vi "Postion Sub.vi"(11 "inpute":string) -> (2 "pos":string, 3 "数字":u32)   [LabVIEW 2015]
panel:
  out "连接的字符串 3":string
  out "子字符串 8":string
  out "子字符串 7":string
  out "子字符串 6":string
  out "连接的字符串 2":string
  out "连接的字符串":string
  out "子字符串 5":string
  out "子字符串 4":string
  out "子字符串 3":string
  out "子字符串 2":string
  out "子字符串":string
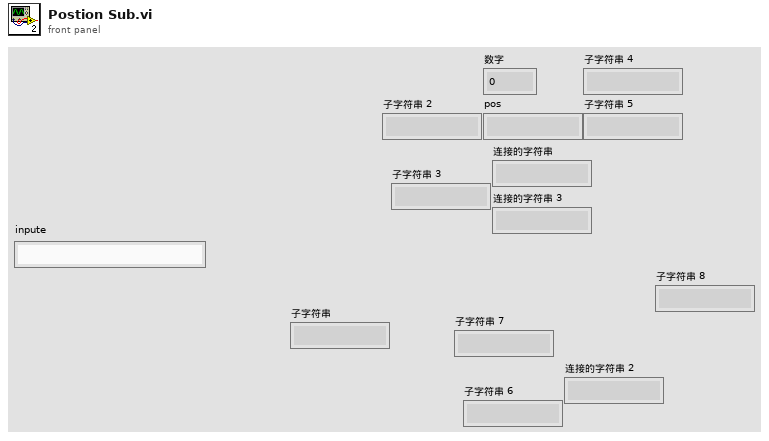
[diagram p1: front panel]
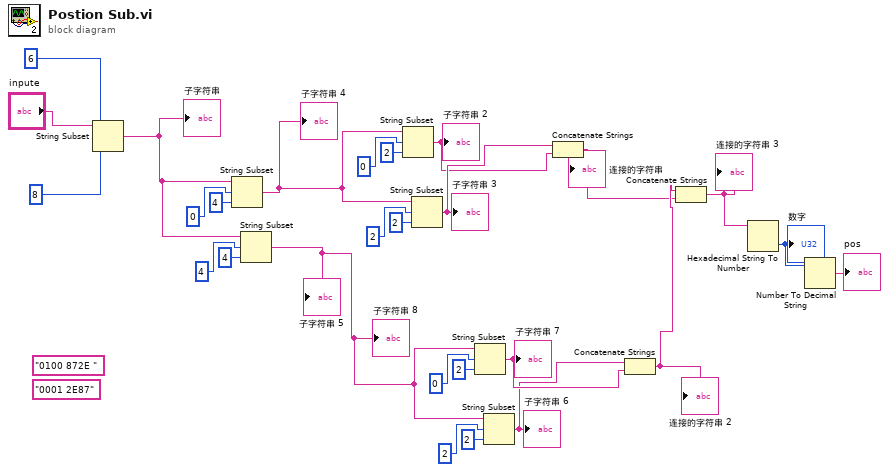
[diagram p0: block diagram]
diagram:
  (unwired) "0001 2E87"
  (unwired) "0100 872E "
  n1 = String Subset(string="inpute", offset (0)=6 ("偏移量(0)"), length (rest)=8 ("长度（剩余）")) -> (substring=w20:string)
  "子字符串" <- w20
  n2 = String Subset(string=w20, offset (0)=0 ("偏移量(0)"), length (rest)=4 ("长度（剩余）")) -> (substring=w13:string)
  "子字符串 4" <- w13
  n3 = String Subset(string=w20, offset (0)=4 ("偏移量(0)"), length (rest)=4 ("长度（剩余）")) -> (substring=w6:string)
  "子字符串 5" <- w6
  "子字符串 8" <- w6
  n4 = String Subset(string=w13, offset (0)=0 ("偏移量(0)"), length (rest)=2 ("长度（剩余）")) -> (substring=w14:string)
  "子字符串 2" <- w14
  n5 = String Subset(string=w13, offset (0)=2 ("偏移量(0)"), length (rest)=2 ("长度（剩余）")) -> (substring=w15:string)
  "子字符串 3" <- w15
  n6 = String Subset(string=w6, offset (0)=0 ("偏移量(0)"), length (rest)=2 ("长度（剩余）")) -> (substring=w12:string)
  "子字符串 7" <- w12
  n7 = String Subset(string=w6, offset (0)=2 ("偏移量(0)"), length (rest)=2 ("长度（剩余）")) -> (substring=w11:string)
  "子字符串 6" <- w11
  n8 = Concatenate Strings(w15, w14) -> (w4:string)
  "连接的字符串" <- w4
  n9 = Concatenate Strings(w11, w12) -> (w5:string)
  "连接的字符串 2" <- w5
  n10 = Concatenate Strings(w5, w4) -> (w1:string)
  "连接的字符串 3" <- w1
  n11 = Hexadecimal String To Number(string=w1) -> (number=w3:u32)  [unwired: 2 in, 1 out]
  "数字" <- w3
  n12 = Number To Decimal String(number=w3) -> (decimal integer string=→"pos":string)  [unwired: 1 in]
